vi "FTW-ScripterStep-Template-Core_Process.vi"(0 "FTW Actor Instance Configuration":string="{\n  \"Identity\": \"ActorName\",\n  \"InboxAddress\": \"inproc://*\",\n  \"LoggerAddress\": \"\",\n  \"My Data\": false,\n  \"Publisher URI\": \"inproc://*\",\n  \"Subscriber URIs\": \"\",\n  \"Refresh Period\": 2\n}", 11 "ErrorIn":errorcluster) -> (15 "Error":errorcluster)   [LabVIEW 2015, in "FTW-ScripterStep-Template-Core.lvclass"]
uses:
  FTW-ScripterStep-Template-Core.lvclass
  source/actor/Message/Base/FTW-Message.lvclass
  FTW-ScripterStep-Template-Core.lvclass/FTW-ScripterStep-Template-Core.ctl
  source/actor/Instance/FTW-ActorInstance.lvclass/FTW-ActorInstance.ctl
  source/actor/JobSequencer/FTW-SEQ-Current.vi
  source/actor/Connector/FTW-ActorConnector.lvclass
  source/actor/Instance/FTW-ActorInstance.lvclass
  source/actor/Message/Request/FTW-Message-IncomingRequest.lvclass
  source/actor/Publisher/FTW-Publisher.lvclass
  source/actor/Subscriber/FTW-Subscriber.lvclass
panel:
  # "#TODO\nhide controls for a GUI"
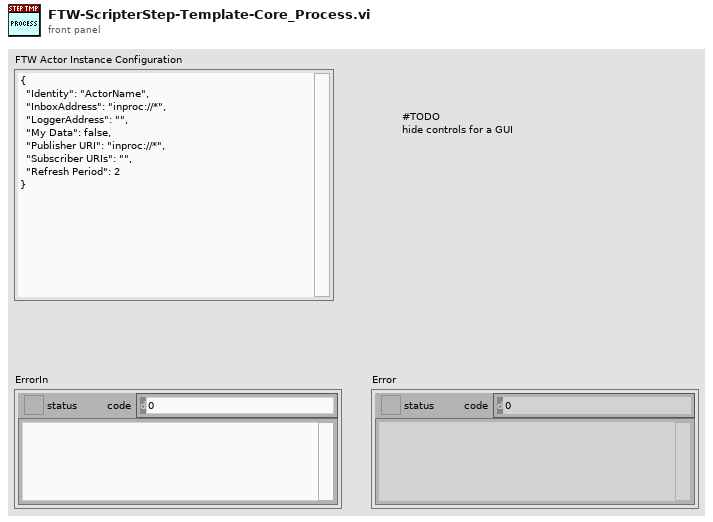
[diagram p1: front panel]
types:
  T1 = cluster{"Incoming Requests":refnum<event-registration>, "Local Messages":refnum<event-registration>, "Subscription":refnum<event-registration>}
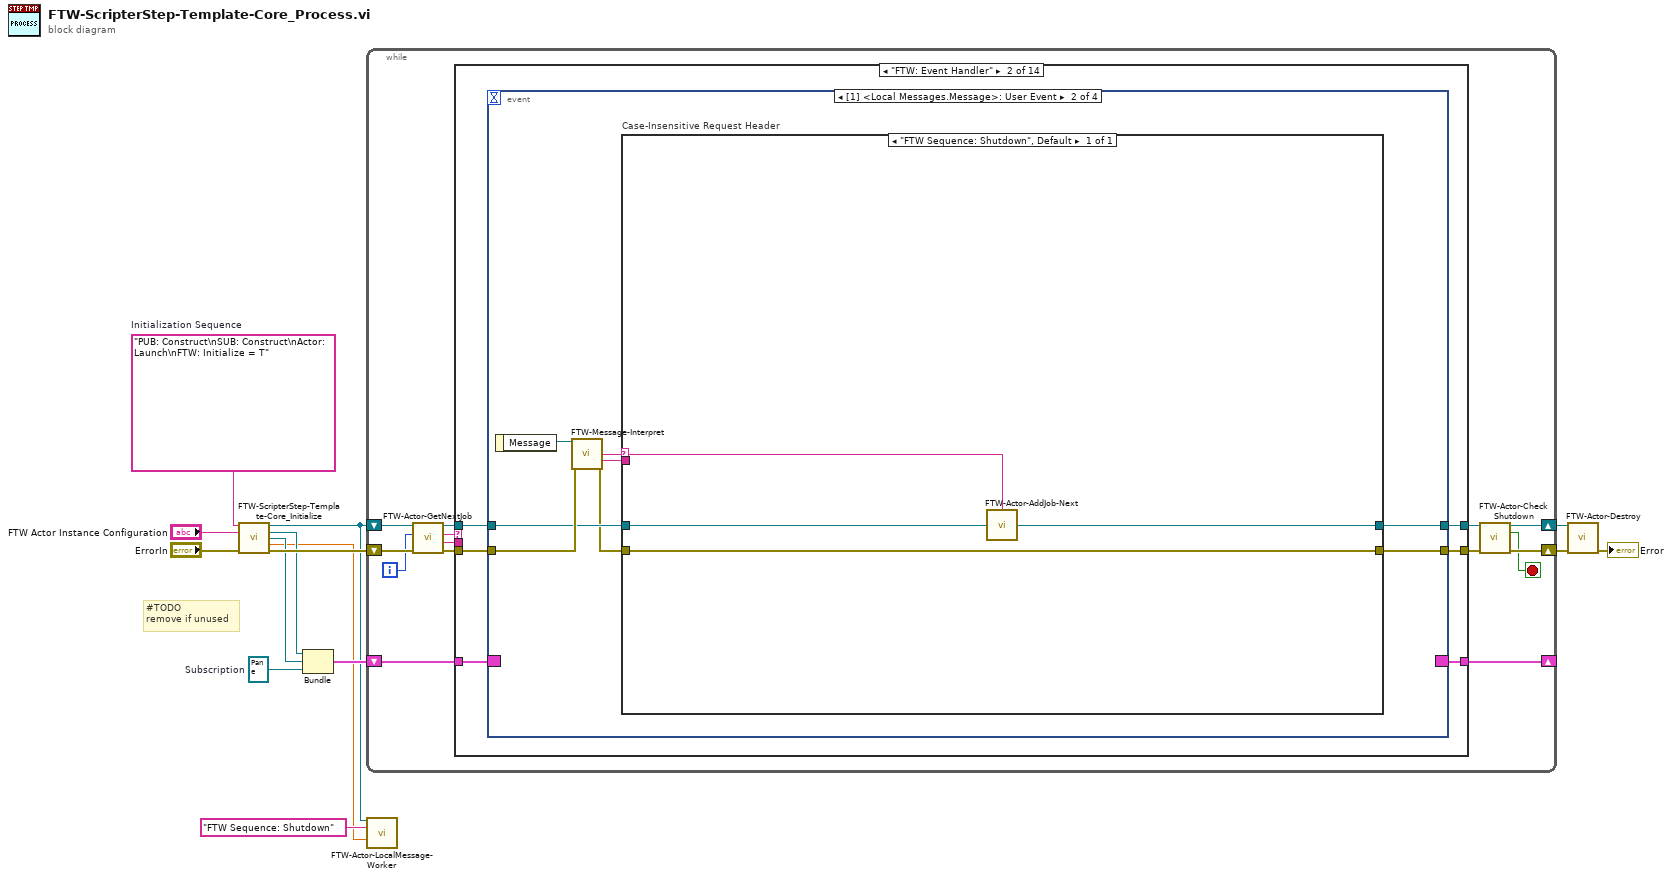
[diagram p0: block diagram]
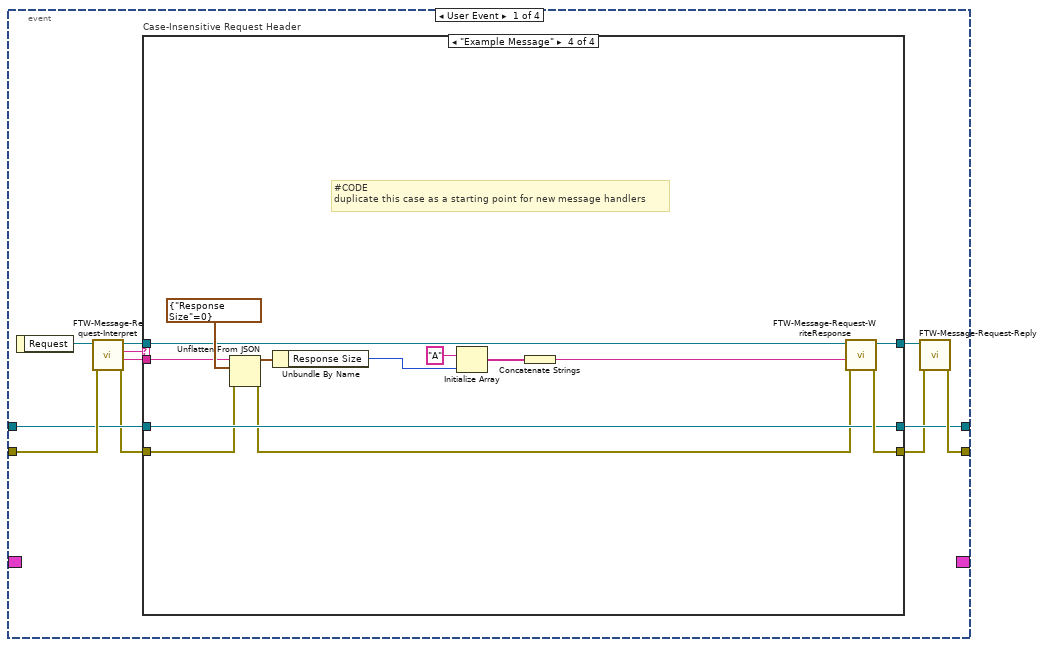
[diagram p3: hidden frame]
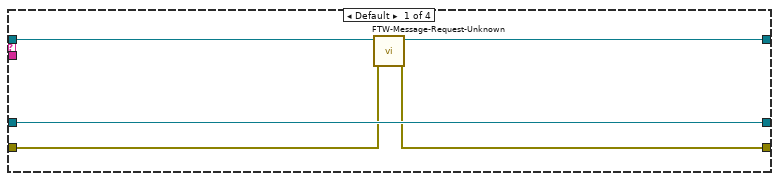
[diagram p4: hidden frame]
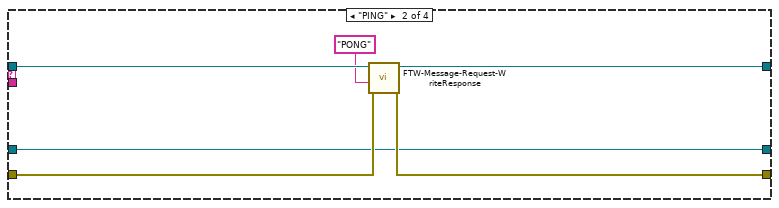
[diagram p5: hidden frame]
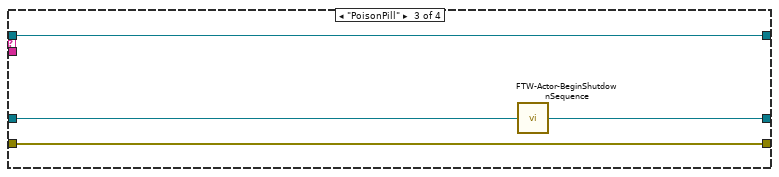
[diagram p6: hidden frame]
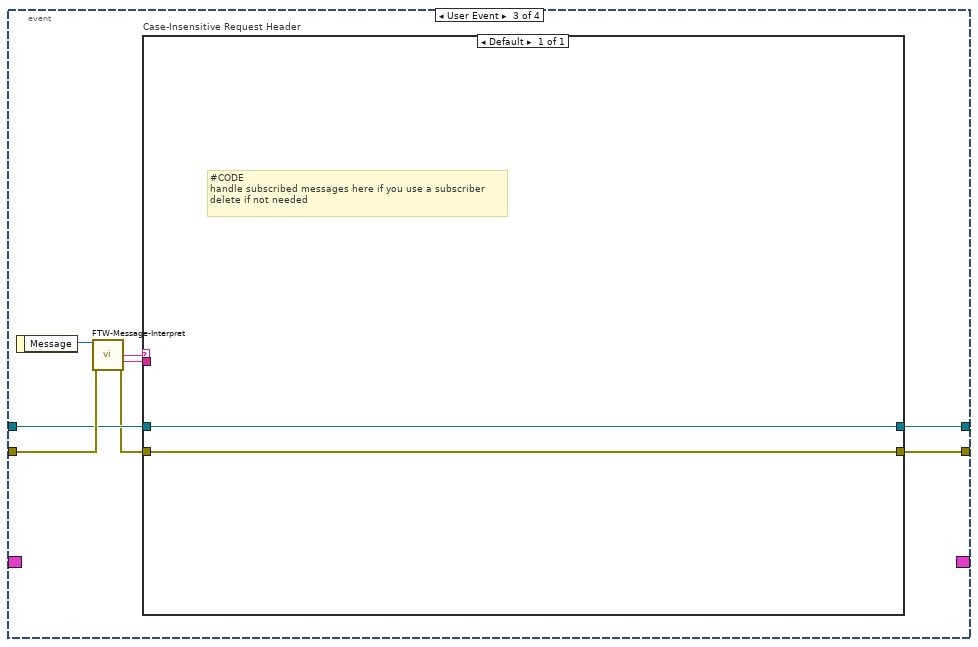
[diagram p7: hidden frame]
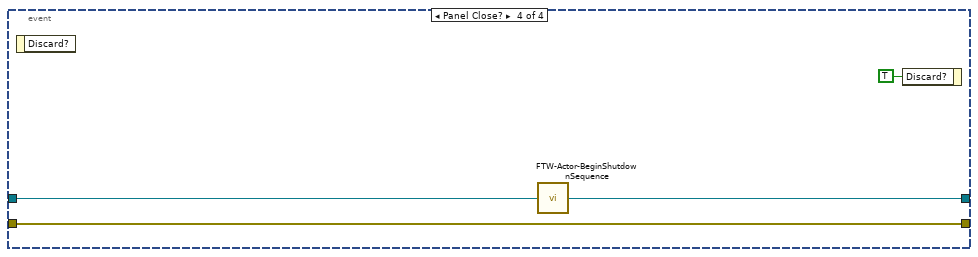
[diagram p8: hidden frame]
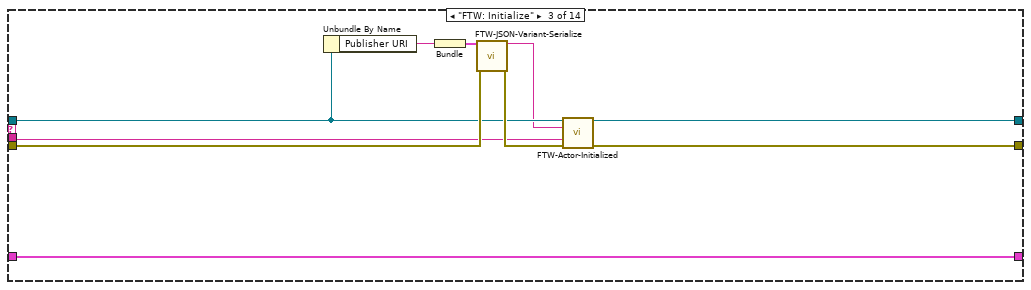
[diagram p9: hidden frame]
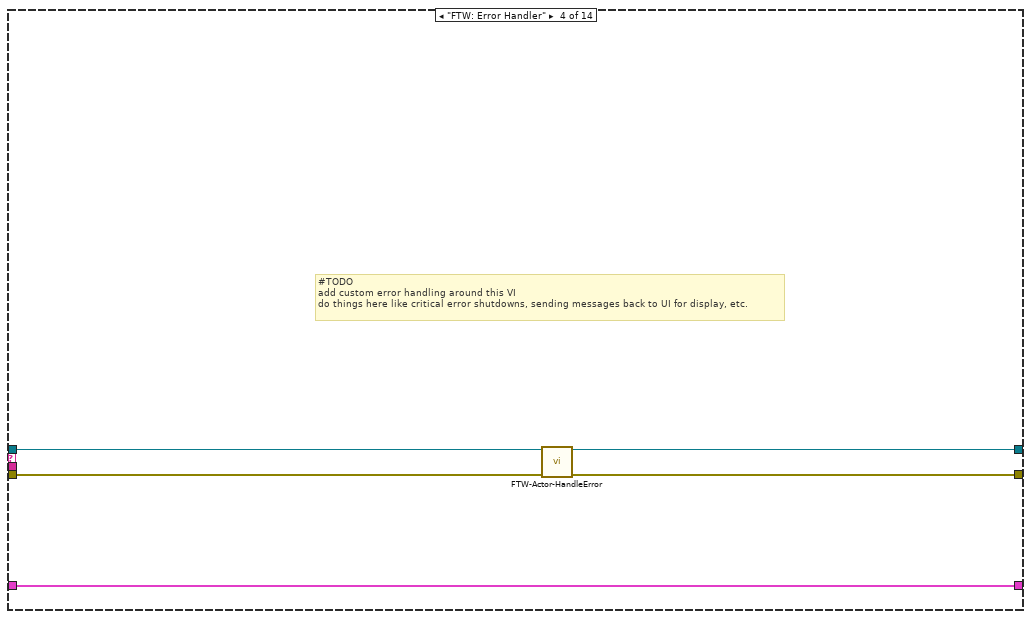
[diagram p10: hidden frame]
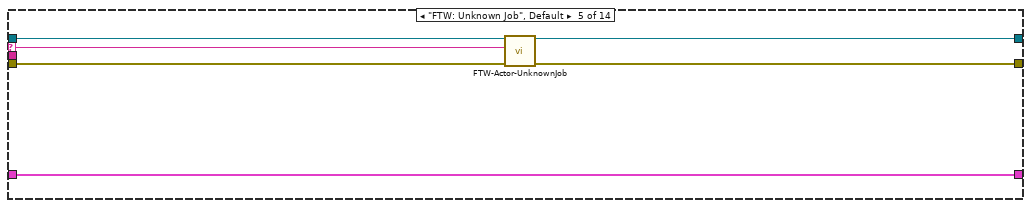
[diagram p11: hidden frame]
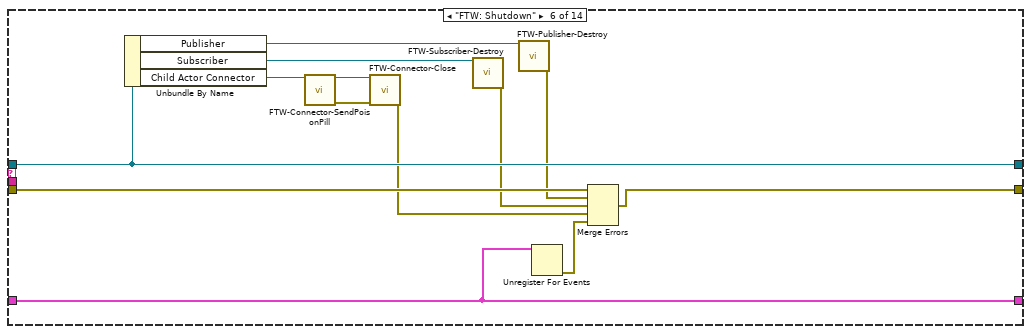
[diagram p12: hidden frame]
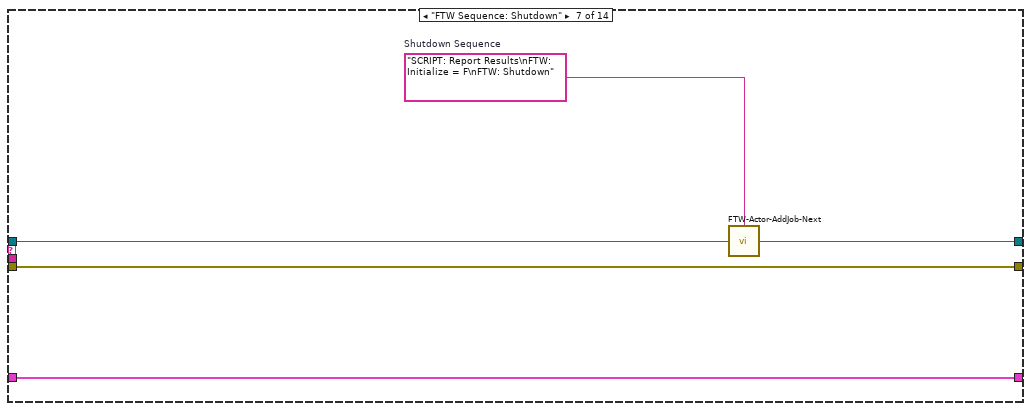
[diagram p13: hidden frame]
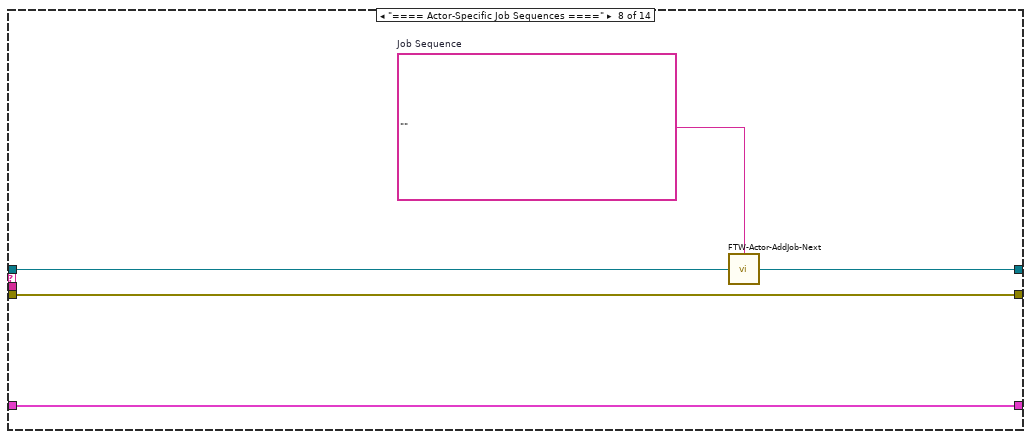
[diagram p14: hidden frame]
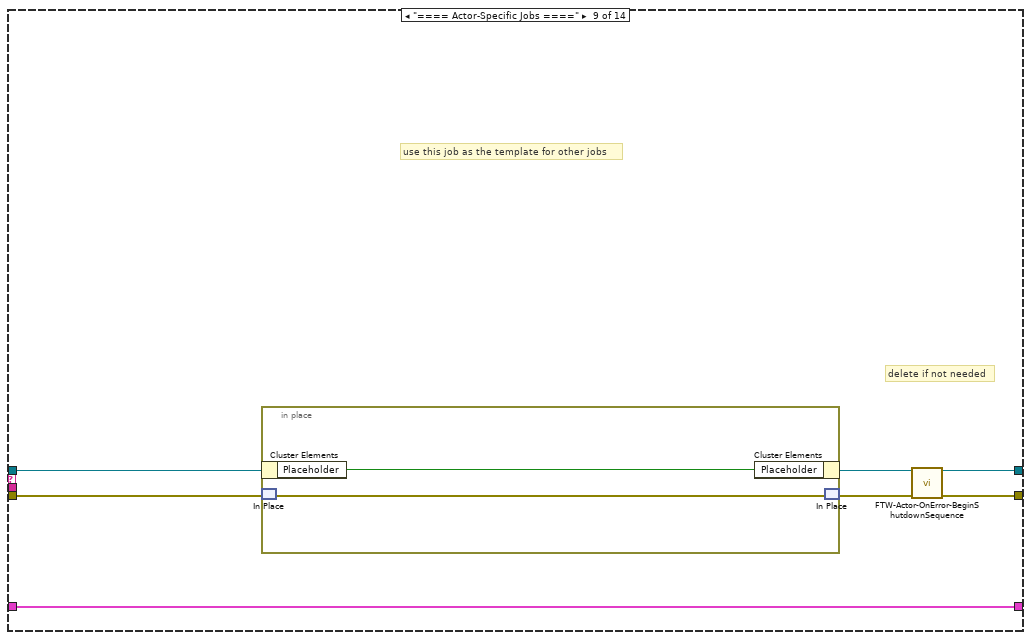
[diagram p15: hidden frame]
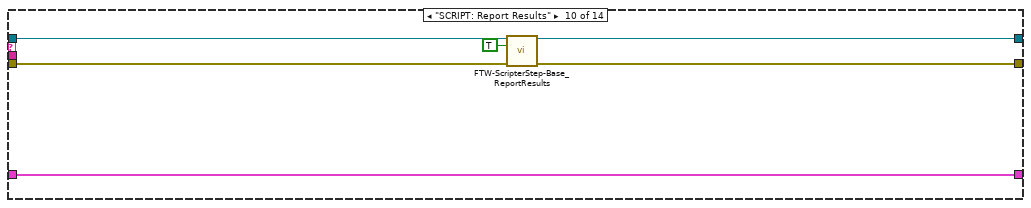
[diagram p16: hidden frame]
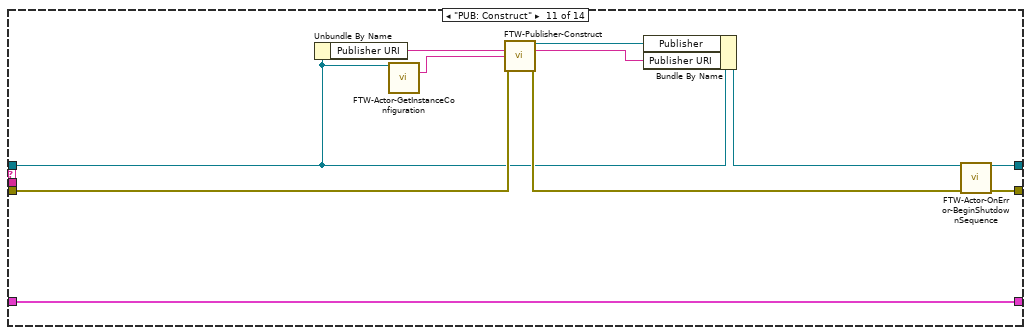
[diagram p17: hidden frame]
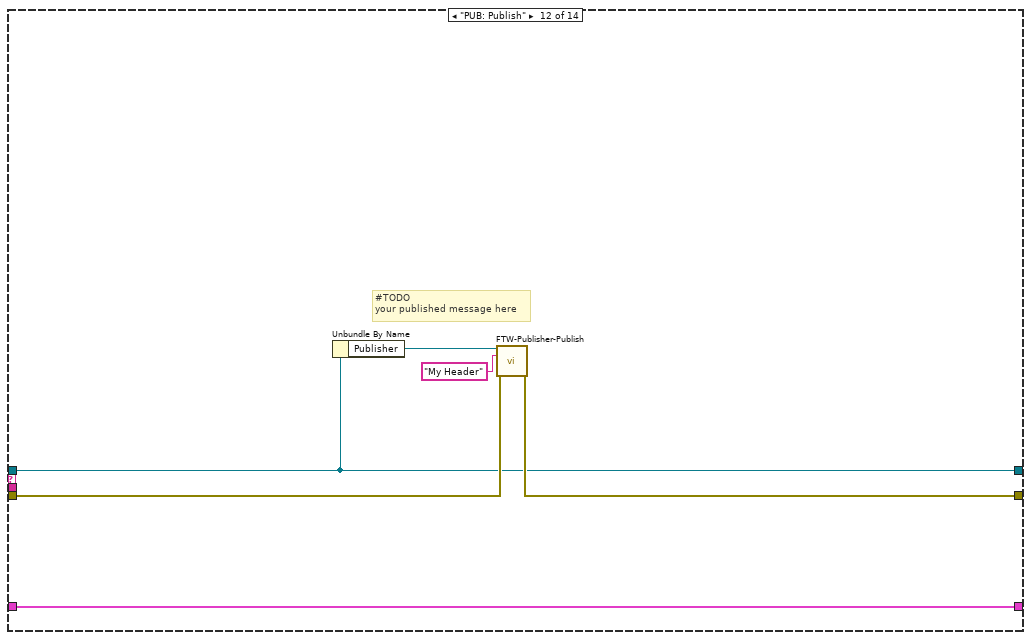
[diagram p18: hidden frame]
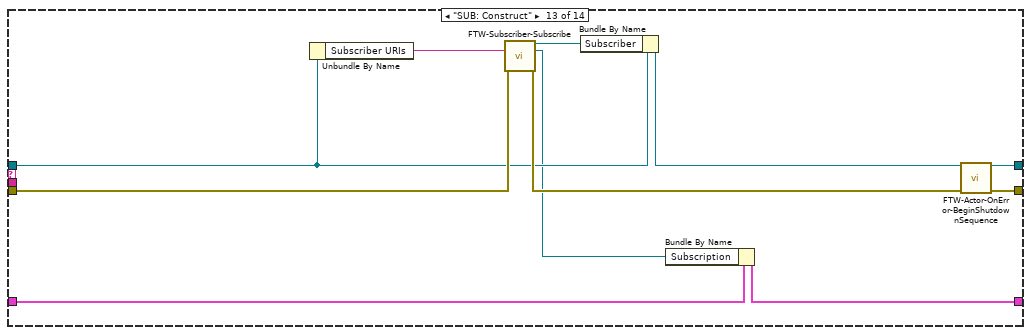
[diagram p19: hidden frame]
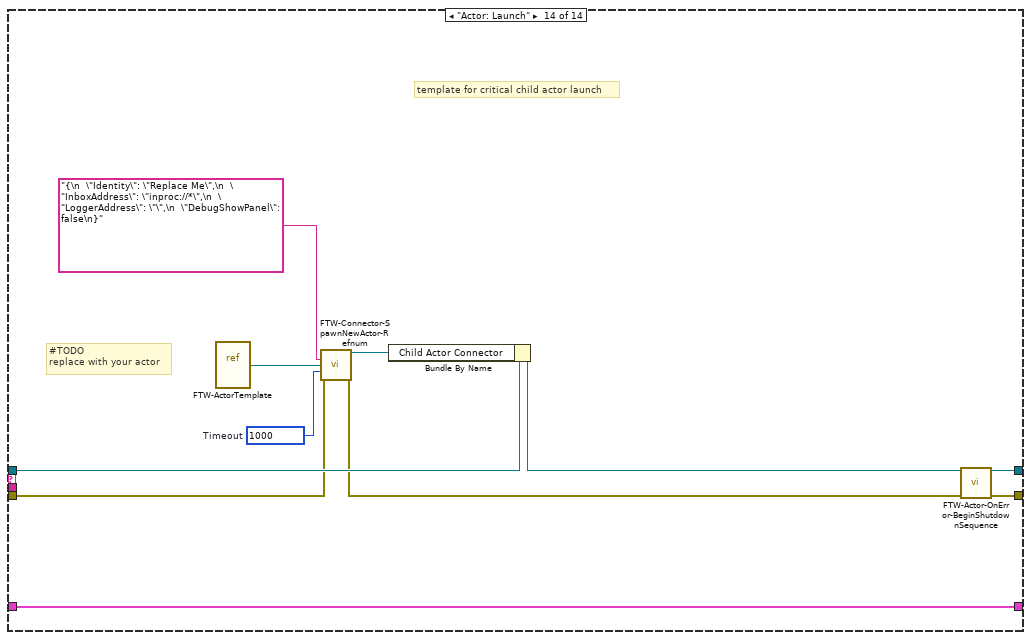
[diagram p20: hidden frame]
diagram:
  w4 = refnum<event-registration> refnum  # Subscription
  w10 = "PUB: Construct\nSUB: Construct\nActor: Launch\nFTW: Initialize = T"  # Initialization Sequence
  # "#TODO\nremove if unused"
  n1 = call "FTW-ScripterStep-Template-Core_Initialize.vi"("Initialization Sequence"=w10, "FTW Actor Instance Configuration"="FTW Actor Instance Configuration", "error in (no error)"="ErrorIn") -> ("Actor Template-Core out"=w2:refnum<class "FTW-ScripterStep-Template-Core.lvclass">, "Incoming Requests"=w6:refnum<event-registration>, "Local Messages"=w5:refnum<event-registration>, "Wait Time"=w1:dbl, "error out"=w11:errorcluster)  [unwired: 8 in]
  n2 = Bundle("Incoming Requests"=w6, "Local Messages"=w5, "Subscription"=w4) -> (w8:T1)  [unwired: 1 in]
  n3 = while {
    shift-right: [w18] -> w13
    shift-left: w11 -> [w25]
    shift-right: [w15] -> _
    shift-left: w8 -> [w28]
    shift-right: [w20] -> w14
    shift-left: w2 -> [w27]
    i -> [w16]
    stop <- w17 stop-if-true
    n4 = call "FTW-Actor-GetNextJob.vi"("error in"=w25, "Jobs Performed"=w16, "FTW Actor Instance"=w27) -> ("error out"=w24:errorcluster, "Job Data"=w22:string, "Job Name"=w23:string, "FTW Actor Instance out"=w26:refnum<class "FTW-ScripterStep-Template-Core.lvclass">)  [unwired: 5 in]
    n5 = case shown="\"FTW: Event Handler\"" w23 {
      selector: w23 -> [_ _ _ _ w118 _ _ _ _ _ _ _ _ _]
      tunnel: [w30 w37 w108 w113 w121 w135 w140 w145 w149 w157 w168 w176 w185 w199] -> w19
      tunnel: w24 -> [w30 w36 w112 w115 w122 w136 w140 w145 w152 w160 w170 w177 w187 w193]
      tunnel: w28 -> [w31 w32 w110 w117 w123 w133 w141 w146 w153 w161 w172 w178 w189 w200]
      tunnel: [w31 w35 w110 w117 w123 w133 w141 w146 w153 w161 w172 w178 w180 w200] -> w15
      tunnel: w22 -> [_ _ w105 _ _ _ _ _ _ _ _ _ _ _]
      tunnel: [w29 w34 w109 w114 w119 w132 w138 w143 w147 w158 w166 w175 w183 w198] -> w21
      tunnel: w26 -> [w29 w33 w107 w116 w120 w132 w139 w144 w150 w159 w163 w175 w181 w197]
      frame "==== Featherweight Framework Jobs ====" {
      }
      frame "FTW: Event Handler" {
        n6 = event shown="[1] <Local Messages.Message>: User Event" {
          selector: w32 -> [_ _ _ _]
          dyn-events: [_ _ _ _] -> w35
          timeout: _ -> [_ _ _ _]
          tunnel: [w47 w79 w91 w101] -> w37
          tunnel: w36 -> [w46 w83 w95 w101]
          tunnel: [w41 w80 w92 w99] -> w34
          tunnel: w33 -> [w45 w82 w94 w100]
          event User Event {
            n7 = event-data() -> ("Request"=w48:refnum<class "FTW-Message-IncomingRequest.lvclass">)  [unwired: 1 in]
            n8 = call "FTW-Message-Request-Interpret.vi"("error in"=w46, "FTW Incoming Request"=w48) -> ("error out"=w44:errorcluster, "Request Body"=w38:string, "Request Header"=w42:string, "FTW Incoming Request out"=w43:refnum<class "FTW-Message-IncomingRequest.lvclass">)  [unwired: 6 in]
            n9 = case "Case-Insensitive Request Header" shown="\"Example Message\"" w42 {
              tunnel: [w51 w57 w62 w76] -> w40
              tunnel: w44 -> [w52 w58 w62 w65]
              tunnel: [w53 w56 w63 w74] -> w41
              tunnel: w45 -> [w53 w56 w61 w74]
              tunnel: w43 -> [w50 w59 w60 w66]
              tunnel: [w49 w55 w60 w75] -> w39
              tunnel: w38 -> [_ _ _ w64]
              frame Default {
                n10 = call "FTW-Message-Request-Unknown.vi"("error in"=w52, "FTW Incoming Request"=w50) -> ("error out"=w51:errorcluster, "FTW Incoming Request Out"=w49:refnum<class "FTW-Message-IncomingRequest.lvclass">)  [unwired: 8 in]
              }
              frame "PING" {
                n11 = call "FTW-Message-Request-WriteResponse.vi"("error in"=w58, "Response Body"="PONG" ("Response Header"), "FTW Incoming Request"=w59) -> ("error out"=w57:errorcluster, "FTW Incoming Request out"=w55:refnum<class "FTW-Message-IncomingRequest.lvclass">)  [unwired: 7 in]
              }
              frame "PoisonPill" {
                n12 = call "FTW-Actor-BeginShutdownSequence.vi"("FTW Actor Instance"=w61) -> ("FTW Actor Instance out"=w63:refnum<class "FTW-ScripterStep-Template-Core.lvclass">)  [unwired: 3 in]
              }
              frame "Example Message" {
                # "#CODE\nduplicate this case as a starting point for new message handlers"
                n13 = Unflatten From JSON(JSON string=w64, type and defaults=cluster{"Response Size":i32} {"Response Size"=0}, error in (no error)=w65) -> (value=w71:cluster{"Response Size":i32}, error out=w73:errorcluster)  [unwired: 4 in]
                n14 = Unbundle By Name(w71) -> ("Response Size"=w70:i32)
                n15 = Initialize Array("A", w70) -> (w68:string[])
                n16 = Concatenate Strings(w68) -> (w67:string)
                n17 = call "FTW-Message-Request-WriteResponse.vi"("error in"=w73, "Response Body"=w67, "FTW Incoming Request"=w66) -> ("error out"=w76:errorcluster, "FTW Incoming Request out"=w75:refnum<class "FTW-Message-IncomingRequest.lvclass">)  [unwired: 7 in]
              }
            }
            n18 = call "FTW-Message-Request-Reply.vi"("FTW: Reply Error"=w40, "FTW Incoming Request"=w39) -> ("error out"=w47:errorcluster)  [unwired: 8 in, 1 out]
          }
          event User Event {
            n19 = event-data() -> ("Message"=w84:refnum<class "FTW-Message.lvclass">)  [unwired: 1 in]
            n20 = call-dynamic "FTW-Message-Interpret.vi"("FTW Message"=w84, "error in"=w83) -> ("Message Header"=w78:string, "Message Body"=w77:string, "error out"=w81:errorcluster)  [unwired: 9 in, 2 out]
            n21 = case "Case-Insensitive Request Header" shown="\"FTW Sequence: Shutdown\", Default" w78 {
              selector: w78 -> [w85]
              tunnel: [w87] -> w79
              tunnel: w81 -> [w87]
              tunnel: [w86] -> w80
              tunnel: w82 -> [w88]
              tunnel: w77 -> [_]
              frame "FTW Sequence: Shutdown", Default {
                n22 = call "FTW-Actor-AddJob-Next.vi"("Add Next in Job Queue"=w85, "FTW Actor Instance"=w88) -> ("FTW Actor Instance out"=w86:refnum<class "FTW-ScripterStep-Template-Core.lvclass">)  [unwired: 2 in]
              }
            }
          }
          event User Event {
            n23 = event-data() -> ("Message"=w96:refnum<class "FTW-Message.lvclass">)  [unwired: 1 in]
            n24 = call-dynamic "FTW-Message-Interpret.vi"("FTW Message"=w96, "error in"=w95) -> ("Message Header"=w90:string, "Message Body"=w89:string, "error out"=w93:errorcluster)  [unwired: 9 in, 2 out]
            n25 = case "Case-Insensitive Request Header" shown="Default" w90 {
              tunnel: [w97] -> w91
              tunnel: w93 -> [w97]
              tunnel: [w98] -> w92
              tunnel: w94 -> [w98]
              tunnel: w89 -> [_]
              frame Default {
                # "#CODE\nhandle subscribed messages here if you use a subscriber\ndelete if not needed"
              }
            }
          }
          event Panel Close? {
            n26 = event-data() -> ()  [unwired: 1 in, 1 out]
            n27 = call "FTW-Actor-BeginShutdownSequence.vi"("FTW Actor Instance"=w100) -> ("FTW Actor Instance out"=w99:refnum<class "FTW-ScripterStep-Template-Core.lvclass">)  [unwired: 3 in]
            n28 = event-data("Discard?"=TRUE) -> ()  [unwired: 1 in, 1 out]
          }
        }
      }
      frame "FTW: Initialize" {
        n29 = Unbundle By Name(w107) -> ("Publisher URI"=w106:string)
        n30 = Bundle("Publisher URI"=w106) -> (w104:cluster{"Publisher URI":string})  [unwired: 1 in]
        n31 = call "FTW-JSON-Variant-Serialize.vi"("Variant"=w104, "error in"=w112) -> ("JSON String"=w103:string, "error out"=w111:errorcluster)  [unwired: 12 in]
        n32 = call-dynamic "FTW-Actor-Initialized.vi"("FTW Actor Instance"=w107, "Initialized Response"=w103, "Positive Init?"=w105, "error in"=w111) -> ("FTW Actor Instance out"=w109:refnum<class "FTW-ScripterStep-Template-Core.lvclass">, "error out"=w108:errorcluster)  [unwired: 10 in]
      }
      frame "FTW: Error Handler" {
        # "#TODO\nadd custom error handling around this VI\ndo things here like critical error shutdowns, sending messages back to UI for display, etc."
        n33 = call-dynamic "FTW-Actor-HandleError.vi"("FTW Actor Instance"=w116, "error in"=w115) -> ("FTW Actor Instance out"=w114:refnum<class "FTW-ScripterStep-Template-Core.lvclass">, "error out"=w113:errorcluster)  [unwired: 10 in, 2 out]
      }
      frame "FTW: Unknown Job", Default {
        n34 = call-dynamic "FTW-Actor-UnknownJob.vi"("FTW Actor Instance"=w120, "Unknown Job"=w118, "error in"=w122) -> ("FTW Actor Instance out"=w119:refnum<class "FTW-ScripterStep-Template-Core.lvclass">, "error out"=w121:errorcluster)  [unwired: 11 in]
      }
      frame "FTW: Shutdown" {
        n35 = Unbundle By Name(w132) -> ("Publisher"=w131:refnum<class "FTW-Publisher.lvclass">, "Subscriber"=w129:refnum<class "FTW-Subscriber.lvclass">, "Child Actor Connector"=w127:refnum<class "FTW-ActorConnector.lvclass">)
        n36 = call-dynamic "FTW-Connector-SendPoisonPill.vi"("FTW Actor Connector"=w127) -> ("FTW Actor Connector out"=w126:refnum<class "FTW-ActorConnector.lvclass">, "error out"=w125:errorcluster)  [unwired: 9 in, 4 out]
        n37 = call-dynamic "FTW-Connector-Close.vi"("FTW Actor Connector"=w126, "error in"=w125) -> ("error out"=w124:errorcluster)  [unwired: 13 in]
        n38 = call "FTW-Subscriber-Destroy.vi"("FTW-Subscription In"=w129) -> ("error out"=w128:errorcluster)  [unwired: 14 in]
        n39 = call "FTW-Publisher-Destroy.vi"("FTW-Publisher In"=w131) -> ("error out"=w130:errorcluster)  [unwired: 14 in]
        n40 = Unregister For Events(event registration refnum=w133) -> (error out=w134:errorcluster)  [unwired: 1 in]
        n41 = Merge Errors(w136, w130, w128, w124, w134) -> (w135:errorcluster)
      }
      frame "FTW Sequence: Shutdown" {
        w137 = "SCRIPT: Report Results\nFTW: Initialize = F\nFTW: Shutdown"  # Shutdown Sequence
        n42 = call "FTW-Actor-AddJob-Next.vi"("Add Next in Job Queue"=w137, "FTW Actor Instance"=w139) -> ("FTW Actor Instance out"=w138:refnum<class "FTW-ScripterStep-Template-Core.lvclass">)  [unwired: 2 in]
      }
      frame "==== Actor-Specific Job Sequences ====" {
        w142 = ""  # Job Sequence
        n43 = call "FTW-Actor-AddJob-Next.vi"("Add Next in Job Queue"=w142, "FTW Actor Instance"=w144) -> ("FTW Actor Instance out"=w143:refnum<class "FTW-ScripterStep-Template-Core.lvclass">)  [unwired: 2 in]
      }
      frame "==== Actor-Specific Jobs ====" {
        # "delete if not needed"
        # "use this job as the template for other jobs"
        n44 = in-place {
          n45 = in-place-cluster #1(w150) -> ("Placeholder"=w154:bool)
          n46 = in-place-match #2(w152) -> (w155:errorcluster)
          n47 = in-place-cluster #1("Placeholder"=w154) -> (w148:refnum<class "FTW-ScripterStep-Template-Core.lvclass">)
          n48 = in-place-match #2(w155) -> (w151:errorcluster)
        }
        n49 = call-dynamic "FTW-Actor-OnError-BeginShutdownSequence.vi"("FTW Actor Instance"=w148, "error in"=w151) -> ("FTW Actor Instance out"=w147:refnum<class "FTW-ScripterStep-Template-Core.lvclass">, "error out"=w149:errorcluster)  [unwired: 12 in]
      }
      frame "SCRIPT: Report Results" {
        n50 = call-dynamic "FTW-ScripterStep-Base_ReportResults.vi"("FTW-ScripterStep-Base In"=w159, "Passed"=TRUE, "error in (no error)"=w160) -> ("FTW-ScripterStep-Base Out"=w158:refnum<class "FTW-ScripterStep-Template-Core.lvclass">, "error out"=w157:errorcluster)  [unwired: 11 in]
      }
      frame "PUB: Construct" {
        n51 = Unbundle By Name(w163) -> ("Publisher URI"=w164:string)
        n52 = call "FTW-Actor-GetInstanceConfiguration.vi"("FTW Actor Instance"=w163) -> ("Identity"=w162:string)  [unwired: 12 in, 2 out]
        n53 = call "FTW-Publisher-Construct.vi"("Address"=w164, "Identity"=w162, "error in"=w170) -> ("FTW-Publisher Out"=w171:refnum<class "FTW-Publisher.lvclass">, "Actual Address"=w165:string, "error out"=w169:errorcluster)  [unwired: 10 in]
        n54 = Bundle By Name(cluster=w163, "Publisher"=w171, "Publisher URI"=w165) -> (w167:refnum<class "FTW-ScripterStep-Template-Core.lvclass">)
        n55 = call-dynamic "FTW-Actor-OnError-BeginShutdownSequence.vi"("FTW Actor Instance"=w167, "error in"=w169) -> ("FTW Actor Instance out"=w166:refnum<class "FTW-ScripterStep-Template-Core.lvclass">, "error out"=w168:errorcluster)  [unwired: 12 in]
      }
      frame "PUB: Publish" {
        # "#TODO\nyour published message here"
        n56 = Unbundle By Name(w175) -> ("Publisher"=w174:refnum<class "FTW-Publisher.lvclass">)
        n57 = call "FTW-Publisher-Publish.vi"("FTW-Publisher In"=w174, "Header"="My Header", "error in"=w177) -> ("error out"=w176:errorcluster)  [unwired: 11 in, 1 out]
      }
      frame "SUB: Construct" {
        n58 = Unbundle By Name(w181) -> ("Subscriber URIs"=w182:string)
        n59 = call "FTW-Subscriber-Subscribe.vi"("Addresses"=w182, "error in"=w187) -> ("FTW-Subscription Out"=w188:refnum<class "FTW-Subscriber.lvclass">, "Subscriber Registration"=w179:refnum<event-registration>, "error out"=w186:errorcluster)  [unwired: 11 in]
        n60 = Bundle By Name(cluster=w181, "Subscriber"=w188) -> (w184:refnum<class "FTW-ScripterStep-Template-Core.lvclass">)
        n61 = Bundle By Name(cluster=w189, "Subscription"=w179) -> (w180:T1)
        n62 = call-dynamic "FTW-Actor-OnError-BeginShutdownSequence.vi"("FTW Actor Instance"=w184, "error in"=w186) -> ("FTW Actor Instance out"=w183:refnum<class "FTW-ScripterStep-Template-Core.lvclass">, "error out"=w185:errorcluster)  [unwired: 12 in]
      }
      frame "Actor: Launch" {
        w196 = 1000  # Timeout
        # "#TODO\nreplace with your actor"
        # "template for critical child actor launch"
        n63 = vi-ref "FTW-ActorTemplate.vi"() -> (w195:refnum<vi>)
        n64 = call "FTW-Connector-SpawnNewActor-Refnum.vi"("Configuration"="{\n  \"Identity\": \"Replace Me\",\n  \"InboxAddress\": \"inproc://*\",\n  \"LoggerAddress\": \"\",\n  \"DebugShowPanel\": false\n}", "Actor VI Refnum"=w195, "Timeout"=w196, "error in"=w193) -> ("FTW Actor Connector"=w190:refnum<class "FTW-ActorConnector.lvclass">, "error out"=w192:errorcluster)  [unwired: 8 in, 2 out]
        n65 = Bundle By Name(cluster=w197, "Child Actor Connector"=w190) -> (w191:refnum<class "FTW-ScripterStep-Template-Core.lvclass">)
        n66 = call-dynamic "FTW-Actor-OnError-BeginShutdownSequence.vi"("FTW Actor Instance"=w191, "error in"=w192) -> ("FTW Actor Instance out"=w198:refnum<class "FTW-ScripterStep-Template-Core.lvclass">, "error out"=w199:errorcluster)  [unwired: 12 in]
      }
    }
    n67 = call "FTW-Actor-CheckShutdown.vi"("FTW Actor Instance"=w21, "error in"=w19) -> ("FTW Actor Instance out"=w20:refnum<class "FTW-ScripterStep-Template-Core.lvclass">, "Shutdown?"=w17:bool, "error out"=w18:errorcluster)  [unwired: 11 in]
  }
  n68 = call-dynamic "FTW-Actor-LocalMessage-Worker.vi"("FTW-ActorInstance In"=w2, "Message Header"="FTW Sequence: Shutdown", "Send Rate"=w1) -> ()  [unwired: 13 in]
  n69 = call-dynamic "FTW-Actor-Destroy.vi"("FTW Actor Instance"=w14, "error in"=w13) -> ("error out"=→"Error":errorcluster)  [unwired: 13 in]
